vi "launcher.vi"(5 "RPM Control":dbl(knob) scale=0.0..6000.0, 6 "Stall":bool, 7 "Period (sec)":dbl) -> (0 "RPM":dbl(knob) scale=0.0..6000.0, 1 "RPM In Tol?":bool, 3 "Motor Output":dbl(slide) scale=0.0..1.0)   [LabVIEW 2012]
uses:
  <vilib>/addons/control/pid/pid.llb/PID (DBL).vi
  <vilib>/addons/control/pid/NI_PID_pid.lvlib
panel:
  in  "Open Loop Div":dbl(knob)=16468.370198348624 scale=0.0..20000.0
  out "State":i32
  in  "Test ?":bool
  in  "RPM Control TEST":dbl(knob) scale=0.0..8000.0
  out "RPM Tolerance":dbl=25.0
  in  "PID Floor":dbl(knob)=1906.027496148522 scale=0.0..2000.0
  out "RPM High":bool
  out "RPM Low":bool
  out "1 RPM":bool
  out "5 RPM":bool
  out "2 RPM":bool
  out "8 RPM":bool
  out "7 RPM":bool
  out "6 RPM":bool
  out "4 RPM":bool
  out "3 RPM":bool
  out "RPM Control Response":cluster{"RPM Control":dbl, dbl}(graph)
  in  "Prop (like D)":dbl(knob)=0.00027400965019870436 scale=0.0..0.01
  in  "Int (like P)":dbl(knob)=0.020206088529440537 scale=0.0..0.1
  in  "Deriv (not used)":dbl(knob) scale=0.0..0.01
  out "PID Output":dbl(graph)
  # "0: Open Loop\n1: Closed Loop"
  # "Bot A: 16,488"
  # "Bot B: 16,488"
  # "2 Feb 2013"
  # "CIM: P=0.000,634, I= 0.020,02"
  # "CIM: P=0.000684, I=0.015, D=0.0"
  # "CIM alt: P=0.000684, I=0.02265, D=0.0"
  # "Bot A Floor : 1900"
  # "Bot B Floor : 1900"
  # "Bot A CIM 19 Feb: P=0.0006344, I=0.02002, D=0.0"
  # "Bot B CIM 19 Feb: P=0.0006344, I=0.02002, D=0.0"
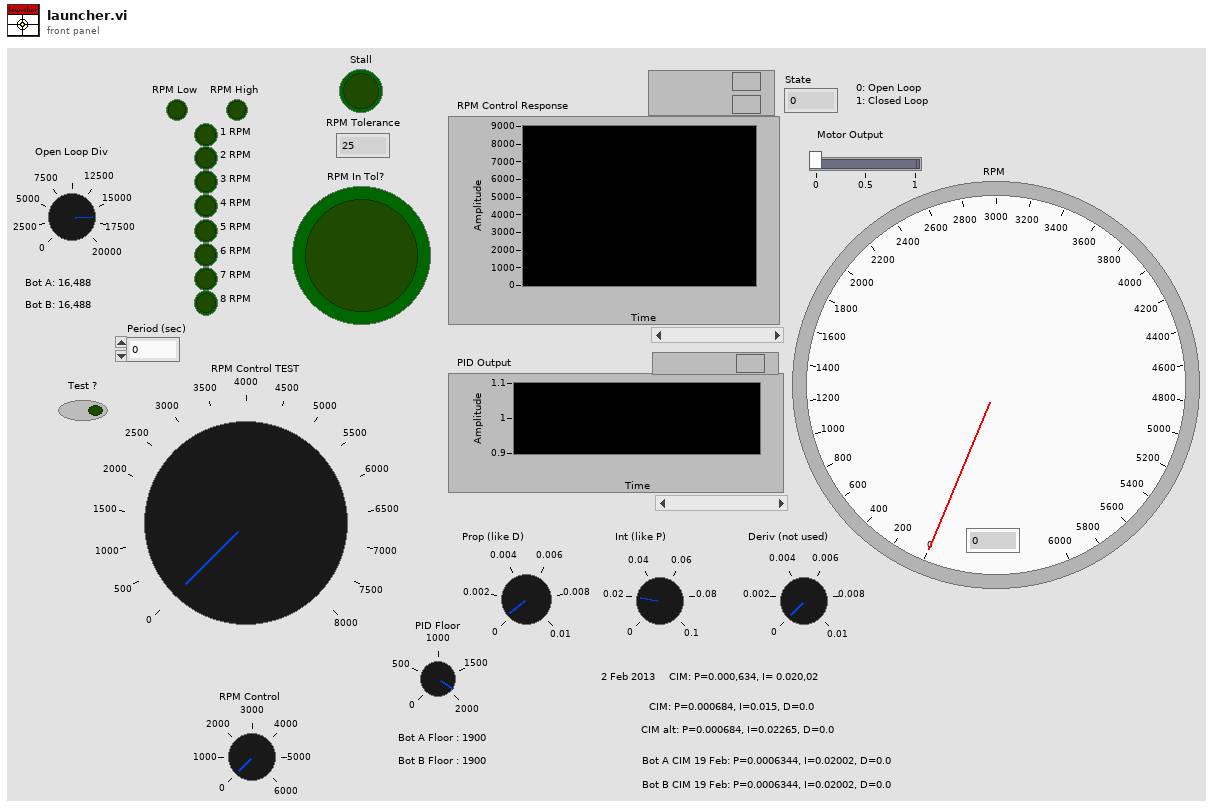
[diagram p1: front panel]
types:
  T1 = cluster{"Prop (like D)":dbl, "Int (like P)":dbl, "Deriv (not used)":dbl}
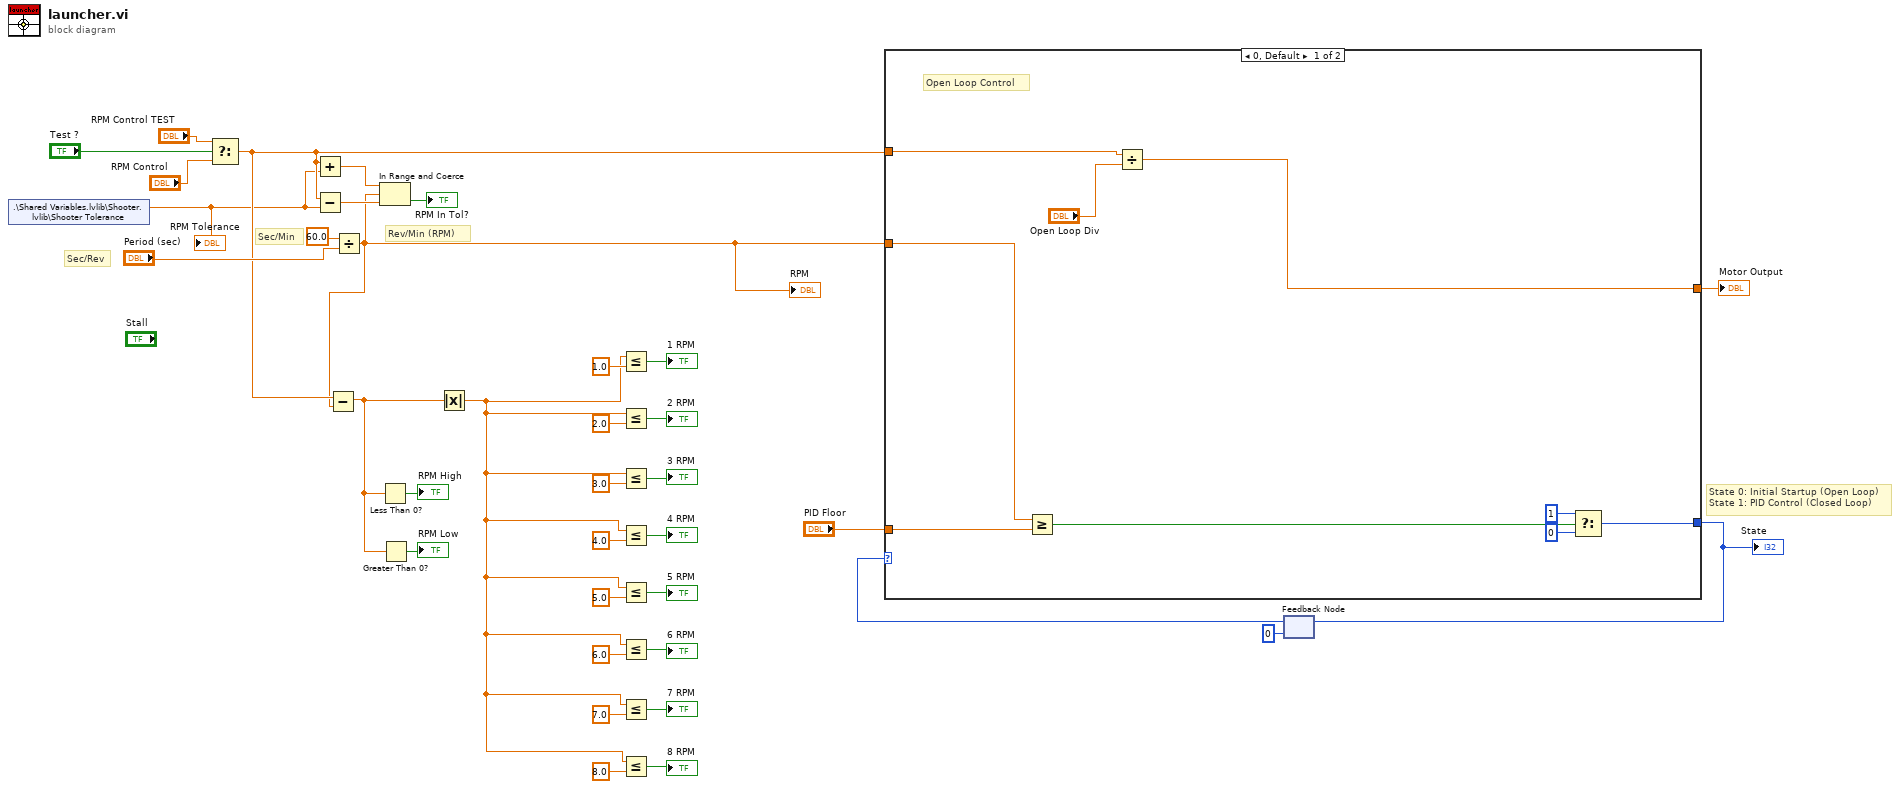
[diagram p0: block diagram]
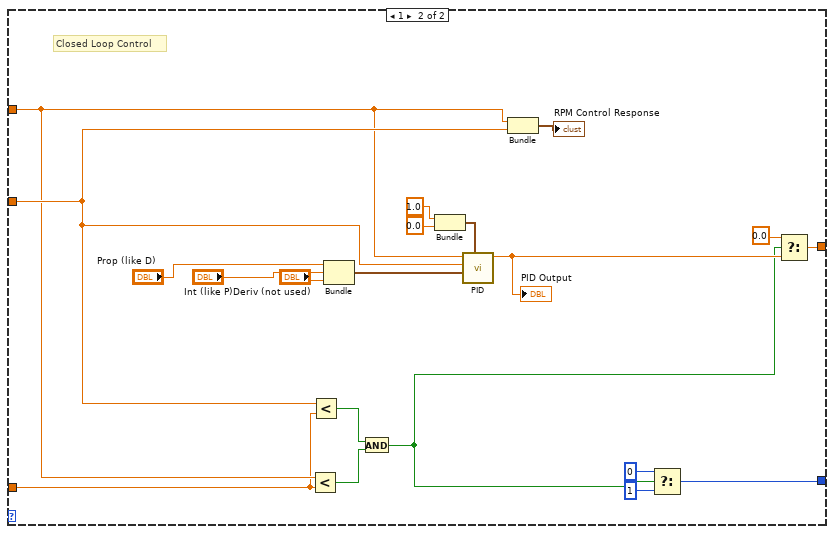
[diagram p2: hidden frame]
diagram:
  # "State 0: Initial Startup (Open Loop)\nState 1: PID Control (Closed Loop)"
  # "Rev/Min (RPM)"
  # "Sec/Rev"
  # "Sec/Min"
  n1 = shared-variable ".\\Shared Variables.lvlib\\Shooter.lvlib\\Shooter Tolerance"() -> (w1:dbl)  [unwired: 1 in, 1 out]
  "RPM Tolerance" <- w1
  n2 = Select(t="RPM Control TEST", s="Test ?", f="RPM Control") -> (s? t:f=w5:dbl)
  n3 = Add(x=w5, y=w1) -> (x+y=w33:dbl)
  n4 = Subtract(x=w5, y=w1) -> (x-y=w34:dbl)
  n5 = Divide(x=60.0 ("y"), y="Period (sec)") -> (x/y=w4:dbl)
  "RPM" <- w4
  n6 = Subtract(x=w5, y=w4) -> (x-y=w13:dbl)
  n7 = In Range and Coerce(upper limit=w33, x=w4, lower limit=w34) -> (In Range?=→"RPM In Tol?":bool)  [unwired: 1 out]
  n8 = Less Than 0?(x=w13) -> (x < 0?=→"RPM High":bool)
  n9 = Greater Than 0?(x=w13) -> (x > 0?=→"RPM Low":bool)
  n10 = Absolute Value(x=w13) -> (abs(x)=w16:dbl)
  n11 = Less Or Equal?(x=w16, y=1.0) -> (x <= y?=→"1 RPM":bool)
  n12 = Less Or Equal?(x=w16, y=2.0) -> (x <= y?=→"2 RPM":bool)
  n13 = Less Or Equal?(x=w16, y=3.0) -> (x <= y?=→"3 RPM":bool)
  n14 = Less Or Equal?(x=w16, y=4.0) -> (x <= y?=→"4 RPM":bool)
  n15 = Less Or Equal?(x=w16, y=5.0) -> (x <= y?=→"5 RPM":bool)
  n16 = Less Or Equal?(x=w16, y=6.0) -> (x <= y?=→"6 RPM":bool)
  n17 = Less Or Equal?(x=w16, y=7.0) -> (x <= y?=→"7 RPM":bool)
  n18 = Less Or Equal?(x=w16, y=8.0) -> (x <= y?=→"8 RPM":bool)
  n19 = feedback #1(0 ("t")) -> (w8:i32)
  n20 = case shown="0, Default" w8 {
    tunnel: [w45 w65] -> w11
    tunnel: w4 -> [w42 w52]
    tunnel: w5 -> [w44 w51]
    tunnel: "PID Floor" -> [w43 w50]
    tunnel: [w38 w46] -> w9
    frame 0, Default {
      # "Open Loop Control"
      n21 = Greater Or Equal?(x=w42, y=w43) -> (x >= y?=w39:bool)
      n22 = Divide(x=w44, y="Open Loop Div") -> (x/y=w45:dbl)
      n23 = Select(t=1, s=w39, f=0) -> (s? t:f=w38:i32)
    }
    frame 1 {
      # "Closed Loop Control"
      n24 = Less?(x=w51, y=w50) -> (x < y?=w53:bool)
      n25 = Less?(x=w52, y=w50) -> (x < y?=w54:bool)
      n26 = Bundle("Prop (like D)"="Prop (like D)", "Int (like P)"="Int (like P)", "Deriv (not used)"="Deriv (not used)") -> (w59:T1)  [unwired: 1 out]
      n27 = And(x=w54, y=w53) -> (x .and. y?=w47:bool)
      n28 = Bundle("x"=1.0, 0.0) -> (w56:cluster{"x":dbl, dbl})  [unwired: 1 out]
      n29 = call-poly <vilib>:"PID.vi"("output range"=w56, "PID gains"=w59, "process variable"=w52, "setpoint"=w51) -> ("output"=w55:dbl)  [unwired: 2 in, 5 out]
      "PID Output" <- w55
      n30 = Bundle("RPM Control"=w51, w52) -> (→"RPM Control Response":cluster{"RPM Control":dbl, dbl})  [unwired: 1 out]
      n31 = Select(t=0, s=w47, f=1) -> (s? t:f=w46:i32)
      n32 = Select(t=0.0, s=w47, f=w55) -> (s? t:f=w65:dbl)
    }
  }
  "Motor Output" <- w11
  "State" <- w9
  n33 = feedback-in #1(w9) -> ()
